vi "Update User.vi"(8 "error In":errorcluster, 9 "Selection":refnum<vi>, 10 "Password":refnum<vi>, 11 "String in":refnum<vi>) -> (0 "error Out":errorcluster, 3 "User Details":T1(array[cluster]))   [LabVIEW 2018]
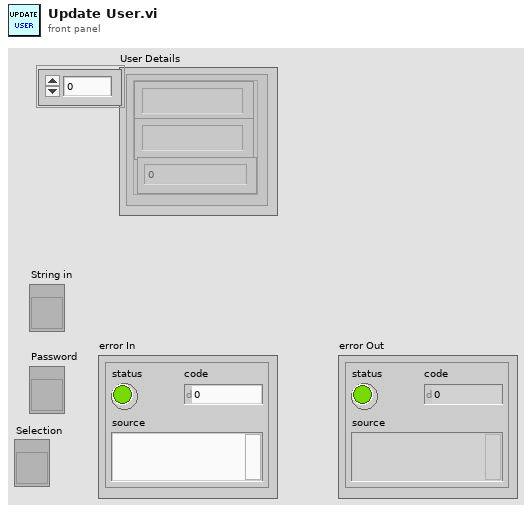
[diagram p1: front panel]
types:
  T1 = cluster{"Default User ":string, "Default Password":string, "Default User Type":u16}[]
  T2 = cluster{"Value":string, "Value":string, "Value":enum16{"VVDN TECH", "Operator", "QA"}}
  T3 = cluster{"Value":string, "Value":string, "Value":enum16{"VVDN TECH", "Operator", "QA"}}[]
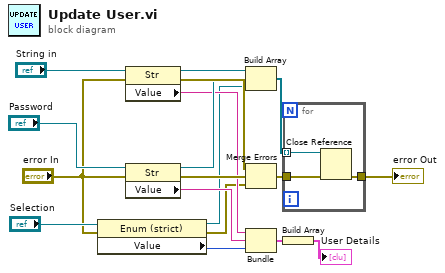
[diagram p0: block diagram]
diagram:
  n1 = property class="Enum (strict)"(reference="Selection", error in="error In") -> (reference out=w3:refnum<vi>, error out=w1:errorcluster, "Value"=w2:enum16{"VVDN TECH", "Operator", "QA"})
  n2 = property class="Str"(reference="String in", error in="error In") -> (reference out=w14:refnum<vi>, error out=w16:errorcluster, "Value"=w9:string)
  n3 = property class="Str"(reference="Password", error in="error In") -> (reference out=w13:refnum<vi>, error out=w15:errorcluster, "Value"=w8:string)
  n4 = Build Array(w14, w13, w3) -> (w12:refnum<vi>[])
  n5 = Merge Errors(w16, w15, w1) -> (w11:errorcluster)
  n6 = Bundle("Value"=w9, "Value"=w8, "Value"=w2) -> (w7:T2)  [unwired: 1 in]
  n7 = for {
    tunnel: w12 -> [w21] mode=indexing
    tunnel: w11 -> [w20]
    tunnel: [w19] -> w10
    n8 = Close Reference(reference=w21, error in (no error)=w20) -> (error out=w19:errorcluster)
  }
  "error Out" <- w10
  n9 = Build Array(w7) -> (→"User Details":T3)
